vi "Enable Disable.vi"(8 "error in (no error)":errorcluster, 11 "Node Ptr":T1 format="%.0x") -> (0 "error out":errorcluster)   [LabVIEW 2020, in "Modbus Master System Explorer.lvlib"]
uses:
  Modbus Master System Explorer.lvlib
  <vilib>/NI VeriStand/Custom Device API/Custom Device Item Ref.ctl
  Shared/Constants.vi
  Shared/Modbus Master Shared.lvlib
  <vilib>/NI VeriStand/Custom Device API/Custom Device API.lvlib
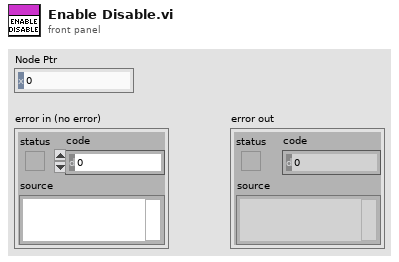
[diagram p1: front panel]
types:
  T1 = typedef "Custom Device API.lvlib/Custom Device Item Ref.ctl" = u64
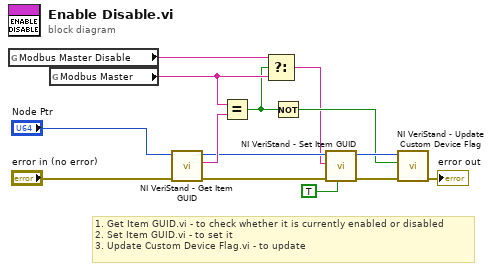
[diagram p0: block diagram]
diagram:
  # "1. Get Item GUID.vi - to check whether it is currently enabled or disabled\n2. Set Item GUID.vi - to set it\n3. Update Custom Device Flag.vi - to update"
  n1 = global read "Constants.vi" "Modbus Master Disable"() -> (w10:string)
  n2 = global read "Constants.vi" "Modbus Master"() -> (w11:string)
  n3 = call <vilib>:"NI VeriStand - Get Item GUID.vi"("error in (no error)"="error in (no error)", "Item Ref in"="Node Ptr") -> ("error out"=w14:errorcluster, "GUID"=w12:string, "Item Ref out"=w8:T1)  [unwired: 7 in]
  n4 = Equal?(x=w11, y=w12) -> (x = y?=w9:bool)
  n5 = Select(t=w10, s=w9, f=w11) -> (s? t:f=w5:string)
  n6 = Not(x=w9) -> (.not. x?=w6:bool)
  n7 = call <vilib>:"NI VeriStand - Set Item GUID.vi"("Refresh System Explorer Tree? (F)"=TRUE, "error in (no error)"=w14, "GUID"=w5, "Item Ref in"=w8) -> ("error out"=w13:errorcluster, "Item Ref out"=w7:T1)  [unwired: 6 in]
  n8 = call <vilib>:"NI VeriStand - Update Custom Device Flag.vi"("error in (no error)"=w13, "Is Custom Device Active?"=w6, "Device Ref in"=w7) -> ("error out"=→"error out":errorcluster)  [unwired: 7 in, 1 out]
